vi "Galvo Module_sync.vi"(5 "sample mode":i32(ring)=10178 items=["Finite Samples"=10178, "Continuous Samples"=10123, "Hardware Timed Single Point"=12522], 7 "Action":T23(ring)=enum."Init: Calc scan pattern", 8 "error in (no error)":errorcluster, 10 "System Parameters":T1={"Optical Parameters"={"Obj. Focal Length [mm]"=45.0, "Scan Lens EFL[mm]"=60.0, "Tube Lens EFL[mm]"=180.0, "Galvo V Range (+/-)"=10.0, "Galvo Max Half Angle [Deg]"=19.0, "Max Galvo Range[%]"=0.0}, "Vibratome"={"Pre Cut Dwell [s]"=0.0, "Blade Frequency [RPM]"=0, "Slice Speed [mm/s]"=0.0, "Post Cut Dwell [s]"=0.0, "Ramp Time [s]"=0.0, "Start X [mm]"=0.0, "Start Y [mm]"=0.0, "Slice Length [mm]"=0.0, "Slice Axis"=enum."Y Axis", "Controller VISA Ref"="COM4", "Blade Frequency [Hz]"=0, "Analog Out Channel"="GalvoCtrl/ao0,GalvoCtrl/ao1", "Pixel Clock Source"="/GalvoCtrl/PFI0", "Vib version"=enum."Vibratome1"}, "Table Stages"={"X Stage"={"Position"=0.0, "Is.Enabled?"=FALSE, "Is.Connected?"=FALSE, "Device SN"="45876539", "AccelerationMaximum"=0.0, "VelocityMaximum"=0.0, "Acceleration"=0.0, "Velocity"=0.0, "waitTimeout (ms)"=0, "Model"=enum."None", "Is.Homed?"=FALSE, "MOVE"=FALSE}, "Y Stage"={"Position"=0.0, "Is.Enabled?"=FALSE, "Is.Connected?"=FALSE, "Device SN"="45876539", "AccelerationMaximum"=0.0, "VelocityMaximum"=0.0, "Acceleration"=0.0, "Velocity"=0.0, "waitTimeout (ms)"=0, "Model"=enum."None", "Is.Homed?"=FALSE, "MOVE"=FALSE}, "Z Stage"={"Position"=0.0, "Is.Enabled?"=FALSE, "Is.Connected?"=FALSE, "Device SN"="45876539", "AccelerationMaximum"=0.0, "VelocityMaximum"=0.0, "Acceleration"=0.0, "Velocity"=0.0, "waitTimeout (ms)"=0, "Model"=enum."None", "Is.Homed?"=FALSE, "MOVE"=FALSE}, "Attenuator"={"Position"=0.0, "Is.Enabled?"=FALSE, "Is.Connected?"=FALSE, "Device SN"="45876539", "AccelerationMaximum"=0.0, "VelocityMaximum"=0.0, "Acceleration"=0.0, "Velocity"=0.0, "waitTimeout (ms)"=0, "Model"=enum."None", "Is.Homed?"=FALSE, "MOVE"=FALSE}}, "Imaging Parameter"={"Raster Scan Direction"=enum."Uni Directional", "Pixel Dwell Time [Clock Cycles]"=1, "Flyback Time [Clock Cycles]"=10, "XY Center [um]"={"X"=1.0, "Y"=1.0}, "Pixel Step Size [um] X"=50.0, "XY Image Size"=enum."256 x 256", "Custom"=TRUE, "Custom Size"={"X"=10, "Y"=10}, "Line Averages"=1, "Pixel Step Size [um] Y"=0.0}, "Galvo HW Parameters"={"Analog Out Channel"="GalvoCtrl/ao0,GalvoCtrl/ao1", "Min Voltage"=-10.0, "Max Voltage"=10.0, "Pixel Clock Source"="/GalvoCtrl/PFI0", "Sample Rate"=1000.0, "Line Clock Out Ch"="GalvoCtrl/port0/line0", "2P ready check"="GalvoCtrl/port0/line0"}, "Alazar parameters"={"Trigger Settings"={"General Trigger Settings"={"Trigger Operation"=0, "Coupling ID"=2, "Range ID"=2, "Delay"=0, "Timeout Ticks"=0, "Mode"=1, "Parameter"=1}, "Trigger Engine 1"={"Trigger Engine"=0, "Source"=2, "Slope"=1, "Level"=140}, "Trigger Engine 2"={"Trigger Engine"=1000, "Source"=4294967295, "Slope"=1, "Level"=2048}}, "Device ID"={"System ID"=1, "Board ID"=1}, "Ch A Input Control"={"Channel"=1, "Coupling"=2, "Range"=10, "Impedance"=2}, "Ch B Input Control"={"Channel"=2, "Coupling"=2, "Range"=10, "Impedance"=2}, "Acq Settings"={"Record Length"=1440, "Offset"=0, "Records Per Buffer"=2048, "Records Count (Records/Acq)"=2147483647, "Window Type"=1, "Footer"=0, "Samples per record"=2048, "Output Format"=257}, "Capture Clock"={"Sample Rate"=100, "Decimation"=0, "Source"=2, "Edge"=0}}, "Mosaic Paramter"={"X Axis"={"Start [mm]"=0.0, "Steps [pts]"=0.0, "End [mm]"=0.0}, "Y Axis"={"Start [mm]"=0.0, "Steps [pts]"=0.0, "End [mm]"=0.0}, "Scan Pattern"=enum."Uni-directional", "Overlap Options"={"Overlap Type"=enum."No Overlap", "Percent Overlap"=0, "Justify"=enum."Start"}}, "Manual Controls"={"Data Path"=path "", "Save parameters"={"start pixel"=45, "#pixels to save"=100}, "Acquisition mode"=enum."Alazar FFT", "PSOCT Channel"=1, "Save data?"=FALSE, "AIP rotation angle"=0.0, "Pause acquisition?"=FALSE, "Outgoing Mail Server (SMTP)"="smtp.gmail.com", "Email"="", "Password"="", "Carrier 1"=enum."Sprint", "phone number 1"="", "Subject"="", "Message"="", "Carrier 2"=enum."Sprint", "phone number 2"="", "Check boundary?"=FALSE, "Threshold"=0.0, "Outputs for GPU FFT"=enum."Amp + Phase diff"}, "Z stage setting"={"first cut height(mm)"=45.85, "slice thickness[um]"=[], "#repetitions"=111, "image thickness(um)"=[], "#cycles per repetition"=0, "First image height(mm)"=2.1, "Block?"=[], "Z0"=0.0, "fixed Z0?"=FALSE}, "Attenuator"={"Power after Objective (recalibrate every 6 month)"=[]}} {"Manual Controls"."PSOCT Channel" items=["A"=1, "B"=2, "A + B"=3, "C"=4, "A + C"=5, "A + B"=6, "D"=8, "A + D"=9, "B + D"=10, "C + D"=12, "A + B + C + D"=15]; "Alazar parameters"."Capture Clock"."Edge" items=["Rising", "Falling"]; "Alazar parameters"."Capture Clock"."Source" items=["Internal"=1, "Fast External"=2, "Medium External"=3, "Slow External"=4, "External AC"=5, "External DC"=6, "External 10MHz"=7]; "Alazar parameters"."Acq Settings"."Output Format" items=["Float Log"=11, "Float Amp"=10, "U16_LOG"=1, "U16_AMP2"=257, "Real"=3, "Imag"=4]; "Alazar parameters"."Acq Settings"."Footer" items=["FOOTER_NONE", "FOOTER_NPT"]; "Alazar parameters"."Acq Settings"."Window Type" items=["DSP_WINDOW_NONE", "DSP_WINDOW_HANNING", "DSP_WINDOW_HAMMING", "DSP_WINDOW_BLACKMAN", "DSP_WINDOW_BLACKMAN_HARRIS", "DSP_WINDOW_BARTLETT"]; "Alazar parameters"."Ch B Input Control"."Channel" items=["A"=1, "B"=2, "C"=4, "D"=8]; "Alazar parameters"."Ch B Input Control"."Coupling" items=["AC"=1, "DC"=2]; "Alazar parameters"."Ch B Input Control"."Range" items=["20 mV"=1, "40 mV"=2, "50 mV"=3, "80 mV"=4, "100 mV"=5, "200 mV"=6, "400 mV"=7, "500 mV"=8, "800 mV"=9, "1 V"=10, "1.25 V"=33, "2 V"=11, "4 V"=12, "5 V"=13, "8 V"=14, "10 V"=15, "20 V"=16]; "Alazar parameters"."Ch B Input Control"."Impedance" items=["1 MOhm"=1, "50 Ohm"=2, ""=0]; "Alazar parameters"."Ch A Input Control"."Channel" items=["A"=1, "B"=2, "C"=4, "D"=8]; "Alazar parameters"."Ch A Input Control"."Coupling" items=["AC"=1, "DC"=2]; "Alazar parameters"."Ch A Input Control"."Range" items=["20 mV"=1, "40 mV"=2, "50 mV"=3, "80 mV"=4, "100 mV"=5, "200 mV"=6, "400 mV"=7, "500 mV"=8, "800 mV"=9, "1 V"=10, "1.25 V"=33, "2 V"=11, "4 V"=12, "5 V"=13, "8 V"=14, "10 V"=15, "20 V"=16]; "Alazar parameters"."Ch A Input Control"."Impedance" items=["1 MOhm"=1, "50 Ohm"=2, ""=0]; "Alazar parameters"."Trigger Settings"."General Trigger Settings"."Trigger Operation" items=["J", "K", "J OR K", "J AND K", "J XOR K", "J AND NOT K", "NOT J AND K"]; "Alazar parameters"."Trigger Settings"."General Trigger Settings"."Coupling ID" items=["AC"=1, "DC"=2]; "Alazar parameters"."Trigger Settings"."General Trigger Settings"."Range ID" items=["5 V", "1 V", "TTL"]; "Alazar parameters"."Trigger Settings"."Trigger Engine 1"."Trigger Engine" items=["J", "K"]; "Alazar parameters"."Trigger Settings"."Trigger Engine 1"."Source" items=["A", "B", "External", "Disable", "C", "D"]; "Alazar parameters"."Trigger Settings"."Trigger Engine 1"."Slope" items=["Positive"=1, "Negative"=2]; "Alazar parameters"."Trigger Settings"."Trigger Engine 2"."Trigger Engine" items=["J", "K"]; "Alazar parameters"."Trigger Settings"."Trigger Engine 2"."Source" items=["A", "B", "External", "Disable", "C", "D"]; "Alazar parameters"."Trigger Settings"."Trigger Engine 2"."Slope" items=["Positive"=1, "Negative"=2]; "Imaging Parameter"."Pixel Step Size [um] Y" min=0.0 max=100.0 step=0.01; "Imaging Parameter"."Line Averages" min=1 max=30 step=1; "Imaging Parameter"."Flyback Time [Clock Cycles]" max=10 step=1; "Imaging Parameter"."Pixel Step Size [um] X" min=0.0 max=100.0 step=0.01; "Imaging Parameter"."Custom Size"."Y" min=1 max=30 step=1; "Imaging Parameter"."Custom Size"."X" min=1 max=30 step=1; "Imaging Parameter"."XY Center [um]"."Y" min=1.0 max=30.0 step=1.0; "Imaging Parameter"."XY Center [um]"."X" min=1.0 max=30.0 step=1.0; "Imaging Parameter"."Pixel Dwell Time [Clock Cycles]" max=10 step=1}) -> (0 "error out":errorcluster, 1 "task done?":bool)   [LabVIEW 2018]
uses:
  Controls/System Parameters.ctl
  Controls/Optical Parameters.ctl
  Controls/Vibratome Parameters.ctl
  type defines/vibratome.ctl
  Controls/Translation Stage Parameters.ctl
  Hardware Mfg/Thorlabs Translation Stages/Controls/Translation Stage Cluster.ctl
  Controls/Translation Stage Types.ctl
  Controls/Imaging Parameters.ctl
  Controls/Scan Direction.ctl
  type defines/Alazar parameters.ctl
  Hardware Mfg/AlazarTech SDK/Controls/General Trigger Settings.ctl
  Hardware Mfg/AlazarTech SDK/Controls/Trigger Engine Controls.ctl
  Hardware Mfg/AlazarTech SDK/Controls/Alazar Device ID.ctl
  Hardware Mfg/AlazarTech SDK/Controls/Channel Input Controls.ctl
  Hardware Mfg/AlazarTech SDK/Controls/Alazar Acquisition Settings.ctl
  Hardware Mfg/AlazarTech SDK/Controls/Clock Controls.ctl
  type defines/Manual Controls.ctl
  type defines/FFT parameters.ctl
  type defines/FFT mode.ctl
  type defines/GPU FFT outputs.ctl
  type defines/Vibratome Param.ctl
  type defines/attenuator.ctl
  <vilib>/DAQmx/write.llb/DAQmx Write (Digital 1D U32 1Chan NSamp).vi
  <vilib>/DAQmx/write.llb/DAQmx Write (Analog 2D DBL NChan NSamp).vi
  <vilib>/DAQmx/create/channels.llb/DAQmx Create Channel (CO-Pulse Generation-Time).vi
  <vilib>/DAQmx/create/channels.llb/DAQmx Create Channel (AO-Voltage-Basic).vi
  <vilib>/DAQmx/configure/timing.llb/DAQmx Timing (Sample Clock).vi
  <vilib>/DAQmx/create/channels.llb/DAQmx Create Channel (DO-Digital Output).vi
  <vilib>/DAQmx/configure/trigger.llb/DAQmx Start Trigger (Digital Edge).vi
  <vilib>/DAQmx/miscellaneous.llb/DAQmx Fill In Error Info.vi
  <resource>/objmgr/daqmx.rc
panel:
  # "X"
  # "X"
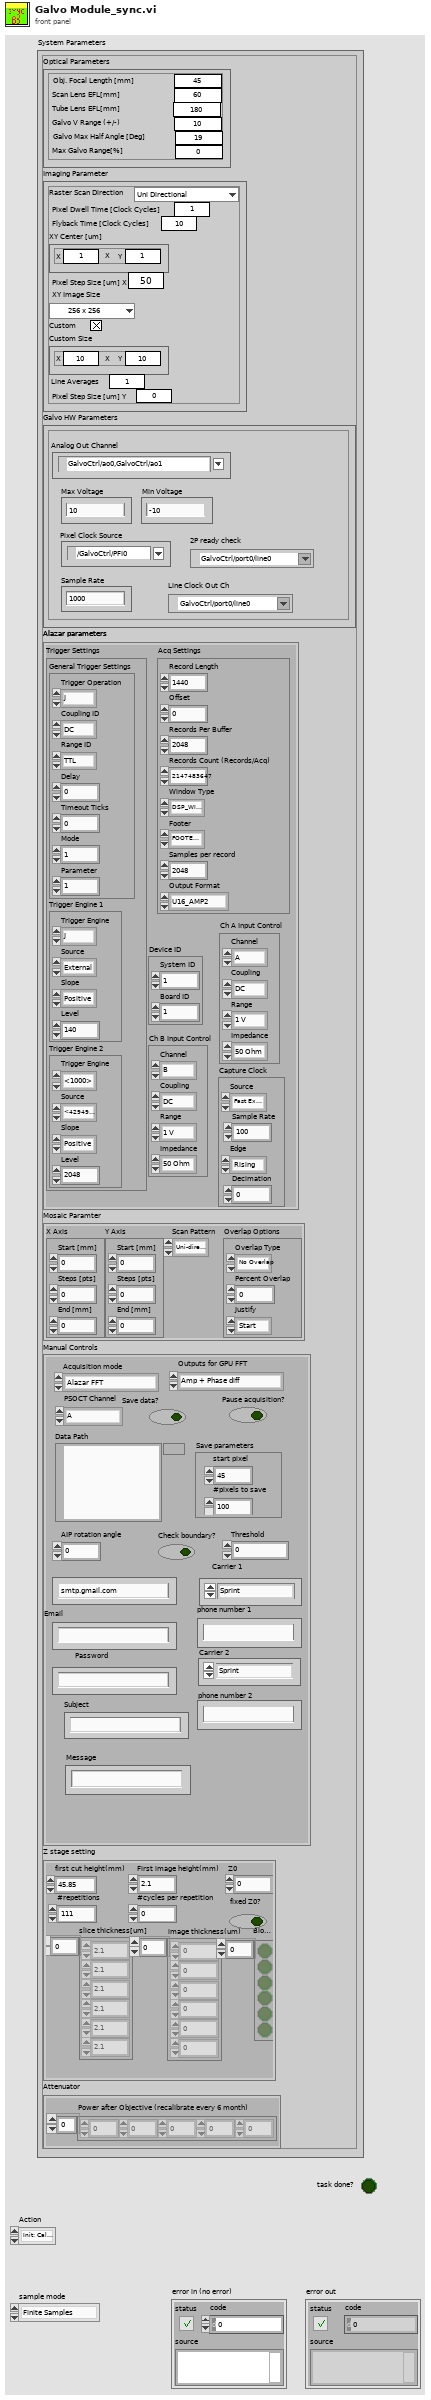
[diagram p1: front panel]
types:
  T1 = typedef "System Parameters.ctl" = cluster{"Optical Parameters":T2, "Vibratome":T3, "Table Stages":T5, "Imaging Parameter":T8, "Galvo HW Parameters":cluster{"Analog Out Channel":tag, "Min Voltage":dbl, "Max Voltage":dbl, "Pixel Clock Source":tag, "Sample Rate":dbl, "Line Clock Out Ch":tag, "2P ready check":tag}, "Alazar parameters":T10, "Mosaic Paramter":cluster{"X Axis":cluster{"Start [mm]":dbl, "Steps [pts]":dbl, "End [mm]":dbl}, "Y Axis":cluster{"Start [mm]":dbl, "Steps [pts]":dbl, "End [mm]":dbl}, "Scan Pattern":enum16{"Uni-directional", "Bi-Directional", "Spiral Out", "Spiral In"}, "Overlap Options":cluster{"Overlap Type":enum16{"No Overlap", "X Only", "Y Only", "X and Y"}, "Percent Overlap":u8, "Justify":enum16{"Start", "Center", "End"}}}, "Manual Controls":T17, "Z stage setting":T21, "Attenuator":T22}
  T2 = typedef "Optical Parameters.ctl" = cluster{"Obj. Focal Length [mm]":dbl, "Scan Lens EFL[mm]":dbl, "Tube Lens EFL[mm]":dbl, "Galvo V Range (+/-)":dbl, "Galvo Max Half Angle [Deg]":dbl, "Max Galvo Range[%]":dbl}
  T3 = typedef "Vibratome Parameters.ctl" = cluster{"Pre Cut Dwell [s]":dbl, "Blade Frequency [RPM]":u16, "Slice Speed [mm/s]":dbl, "Post Cut Dwell [s]":dbl, "Ramp Time [s]":dbl, "Start X [mm]":dbl, "Start Y [mm]":dbl, "Slice Length [mm]":dbl, "Slice Axis":enum16{"X Axis", "Y Axis", "Z Axis"}, "Controller VISA Ref":refnum<visa-resource-name>, "Blade Frequency [Hz]":u16, "Analog Out Channel":tag, "Pixel Clock Source":tag, "Vib version":T4}
  T4 = typedef "vibratome.ctl" = enum16{"Vibratome1", "Vibratome3"}
  T5 = typedef "Translation Stage Parameters.ctl" = cluster{"X Stage":T6, "Y Stage":T6, "Z Stage":T6, "Attenuator":T6}
  T6 = typedef "Translation Stage Cluster.ctl" = cluster{"Position":dbl, "Is.Enabled?":bool, "Is.Connected?":bool, "Device SN":string, "AccelerationMaximum":dbl, "VelocityMaximum":dbl, "Acceleration":dbl, "Velocity":dbl, "waitTimeout (ms)":i32, "Model":T7, "Is.Homed?":bool, "MOVE":bool}
  T7 = typedef "Translation Stage Types.ctl" = enum16{"None", "Thorlabs LTS", "Thorlabs MLJ"}
  T8 = typedef "Imaging Parameters.ctl" = cluster{"Raster Scan Direction":T9, "Pixel Dwell Time [Clock Cycles]":u16, "Flyback Time [Clock Cycles]":u16, "XY Center [um]":cluster{"X":dbl, "Y":dbl}, "Pixel Step Size [um] X":dbl, "XY Image Size":enum16{"32 x 32", "64 x 64", "128 x 128", "256 x 256", "512 x 512", "1024 x 1024", "2048 x 2048"}, "Custom":bool, "Custom Size":cluster{"X":u16, "Y":u16}, "Line Averages":u8, "Pixel Step Size [um] Y":dbl}
  T9 = typedef "Scan Direction.ctl" = enum16{"Uni Directional", "Bi Directional", "None"}
  T10 = typedef "Alazar parameters.ctl" = cluster{"Trigger Settings":cluster{"General Trigger Settings":T11, "Trigger Engine 1":T12, "Trigger Engine 2":T12}, "Device ID":T13, "Ch A Input Control":T14, "Ch B Input Control":T14, "Acq Settings":T15, "Capture Clock":T16}
  T11 = typedef "General Trigger Settings.ctl" = cluster{"Trigger Operation":u32, "Coupling ID":u32, "Range ID":u32, "Delay":u32, "Timeout Ticks":u32, "Mode":u32, "Parameter":u32}
  T12 = typedef "Trigger Engine Controls.ctl" = cluster{"Trigger Engine":u32, "Source":u32, "Slope":u32, "Level":u32}
  T13 = typedef "Alazar Device ID.ctl" = cluster{"System ID":u32, "Board ID":u32}
  T14 = typedef "Channel Input Controls.ctl" = cluster{"Channel":u8, "Coupling":u32, "Range":u32, "Impedance":u32}
  T15 = typedef "Alazar Acquisition Settings.ctl" = cluster{"Record Length":u32, "Offset":u32, "Records Per Buffer":u32, "Records Count (Records/Acq)":u32, "Window Type":u32, "Footer":u32, "Samples per record":u32, "Output Format":u32}
  T16 = typedef "Clock Controls.ctl" = cluster{"Sample Rate":u32, "Decimation":u32, "Source":u32, "Edge":u32}
  T17 = typedef "Manual Controls.ctl" = cluster{"Data Path":path, "Save parameters":T18, "Acquisition mode":T19, "PSOCT Channel":u32, "Save data?":bool, "AIP rotation angle":dbl, "Pause acquisition?":bool, "Outgoing Mail Server (SMTP)":string, "Email":string, "Password":string, "Carrier 1":enum16{"T-Mobile", "AT&T", "Verizon", "Sprint"}, "phone number 1":string, "Subject":string, "Message":string, "Carrier 2":enum16{"T-Mobile", "AT&T", "Verizon", "Sprint"}, "phone number 2":string, "Check boundary?":bool, "Threshold":sgl, "Outputs for GPU FFT":T20}
  T18 = typedef "FFT parameters.ctl" = cluster{"start pixel":i32, "#pixels to save":i32}
  T19 = typedef "FFT mode.ctl" = enum16{"ThorOCT B line", "ThorOCT Spectral", "ThorOCT FFT", "Alazar B line", "Alazar FFT", "GPU FFT", "Alazar Spectral", "Simulation", "auto adjust focus", "Save all"}
  T20 = typedef "GPU FFT outputs.ctl" = enum16{"Amp + Phase diff", "Amp + Phase", "Amp only"}
  T21 = typedef "Vibratome Param.ctl" = cluster{"first cut height(mm)":dbl, "slice thickness[um]":dbl[], "#repetitions":u16, "image thickness(um)":dbl[], "#cycles per repetition":u16, "First image height(mm)":dbl, "Block?":bool[], "Z0":dbl, "fixed Z0?":bool}
  T22 = typedef "attenuator.ctl" = cluster{"Power after Objective (recalibrate every 6 month)":dbl[]}
  T23 = enum16{"Configure channels", "Write Scan Pattern", "Start Galvo Task", "Is Task Done?", "Stop Galvo", "Uninit", "Init: Calc scan pattern"}
  T24 = cluster{"Analog Out Channel":tag, "Min Voltage":dbl, "Max Voltage":dbl, "Pixel Clock Source":tag, "Sample Rate":dbl, "Line Clock Out Ch":tag, "2P ready check":tag}
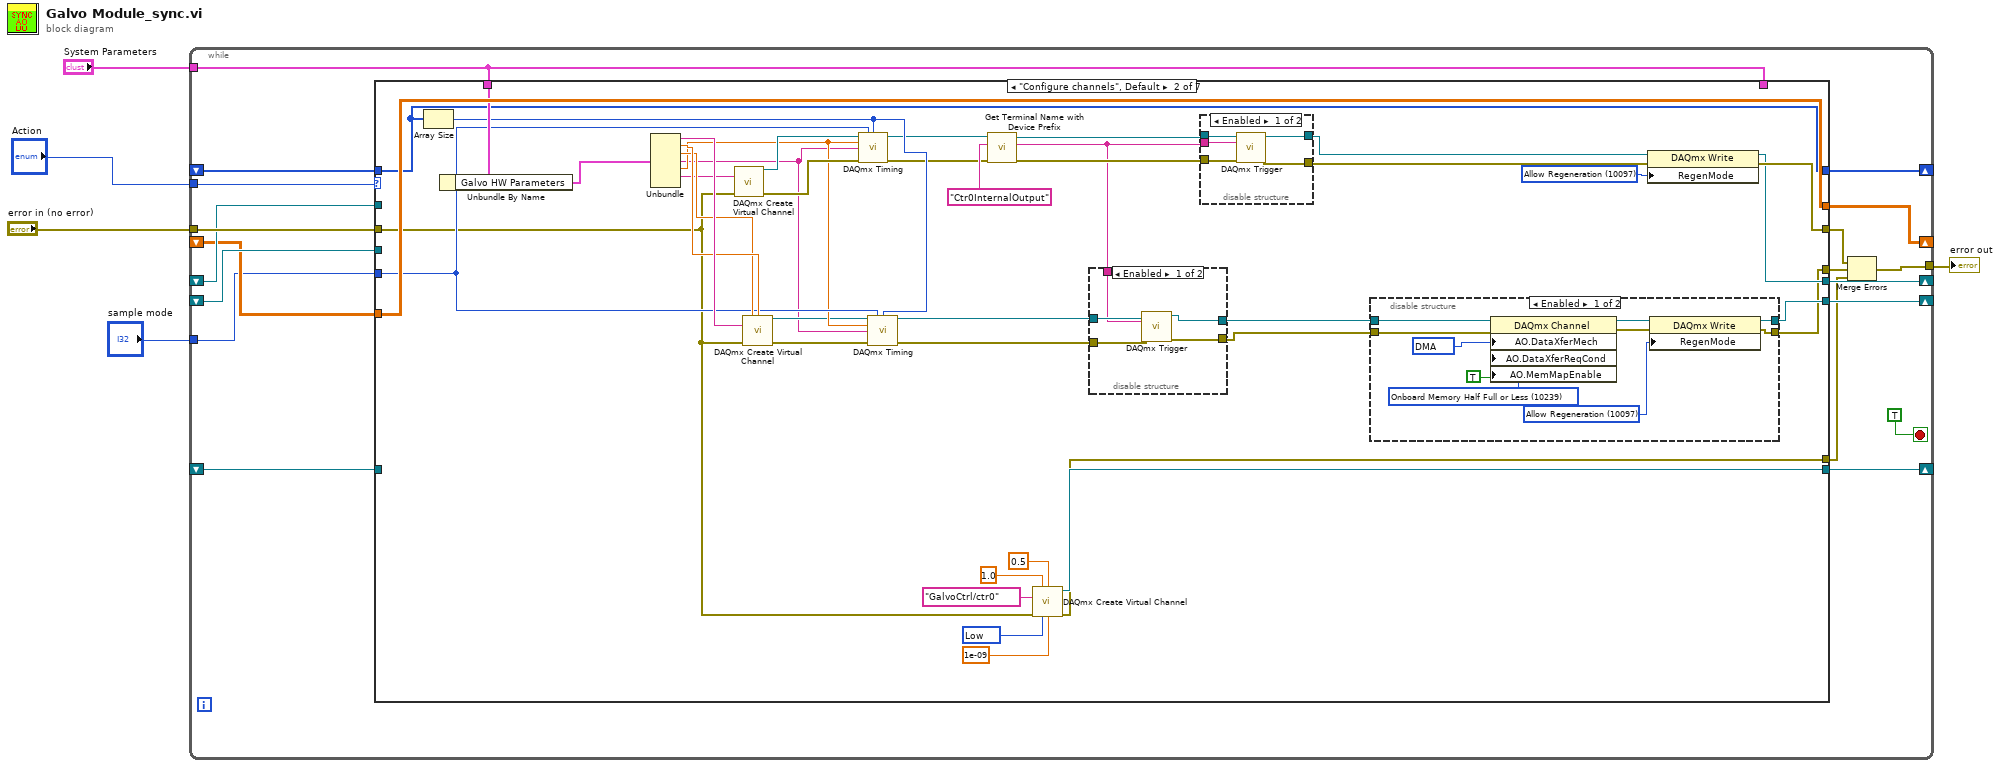
[diagram p0: block diagram]
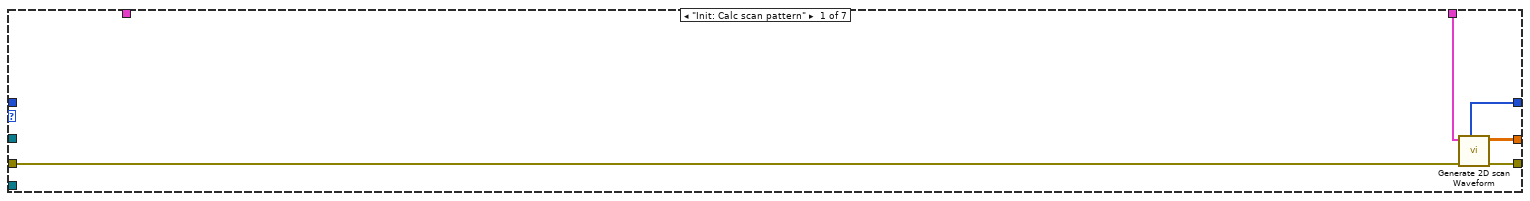
[diagram p2: hidden frame]
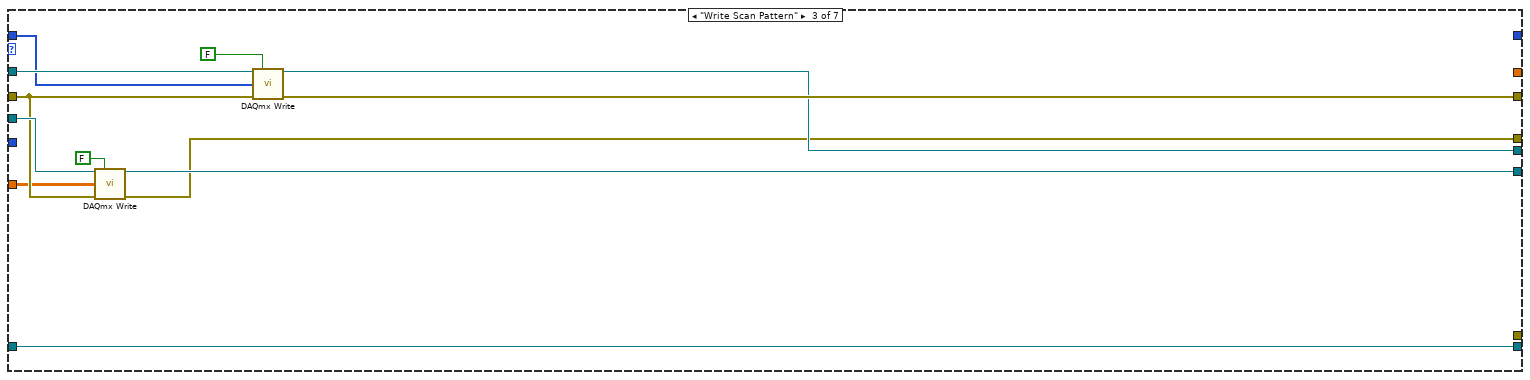
[diagram p6: hidden frame]
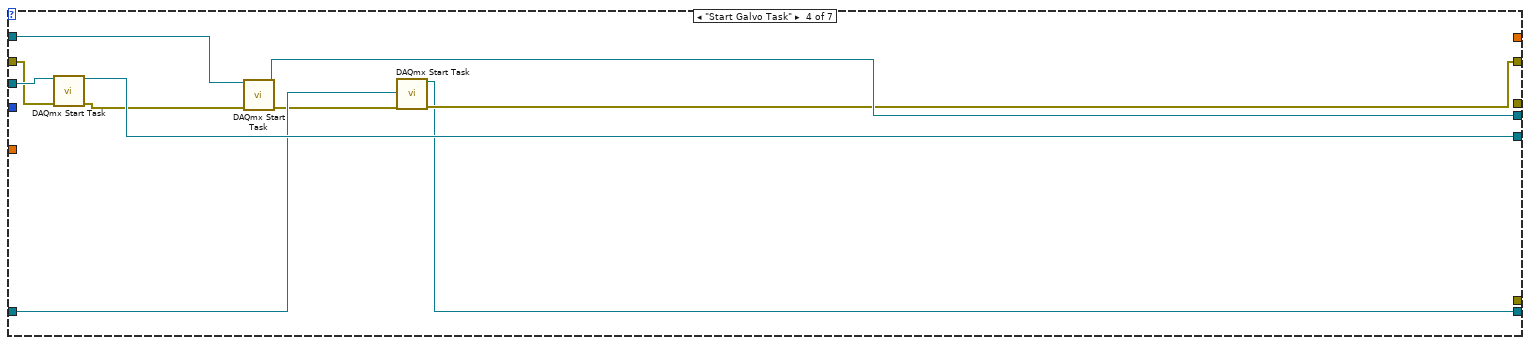
[diagram p7: hidden frame]
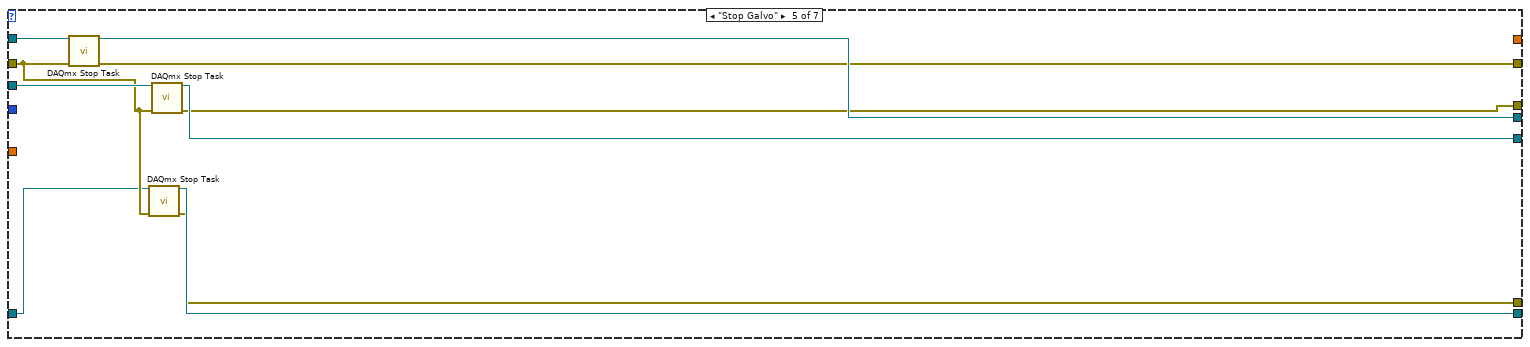
[diagram p8: hidden frame]
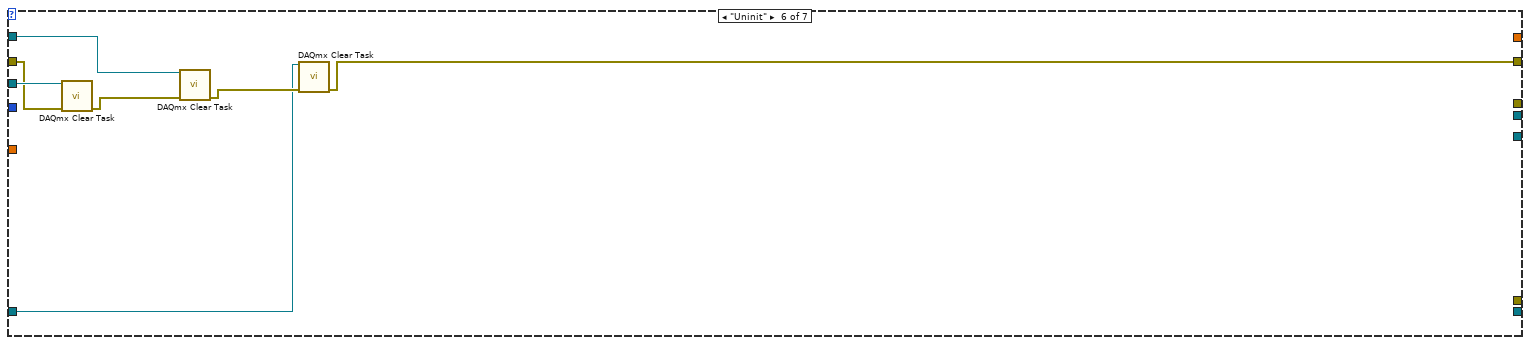
[diagram p9: hidden frame]
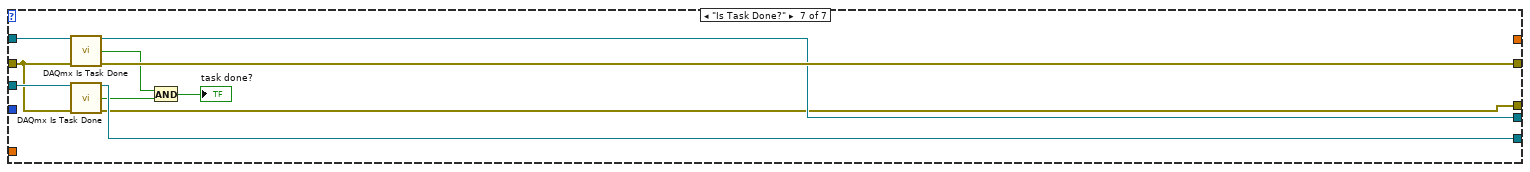
[diagram p10: hidden frame]
diagram:
  n1 = while {
    tunnel: "Action" -> [w24]
    shift-right: [w23] -> _
    shift-left: _ -> [w22]
    tunnel: [w19] -> w4
    tunnel: "error in (no error)" -> [w21]
    shift-right: [w17] -> _
    shift-left: _ -> [w16]
    shift-right: [w15] -> _
    shift-left: _ -> [w14]
    tunnel: "sample mode" -> [w13]
    tunnel: "System Parameters" -> [w11]
    shift-right: [w10] -> _
    shift-left: _ -> [w9]
    shift-right: [w8] -> _
    shift-left: _ -> [w7]
    stop <- TRUE stop-if-true
    n2 = case shown="\"Configure channels\", Default" w24 {
      tunnel: [_ w67 w102 w117 w127 _ w144] -> w23
      tunnel: w22 -> [_ _ w108 w118 w128 w135 w145]
      tunnel: w21 -> [w27 w46 w107 w114 w122 w133 w136]
      tunnel: [w28 w63 w106 w110 w124 w130 w141] -> w18
      tunnel: [_ w62 w104 w115 w125 _ w138] -> w17
      tunnel: w16 -> [_ _ w103 w116 w126 w134 w142]
      tunnel: [w29 w61 _ _ _ _ _] -> w15
      tunnel: w14 -> [_ w61 w101 _ _ _ _]
      tunnel: w13 -> [_ w57 _ _ _ _ _]
      tunnel: [_ w60 w100 _ w123 _ w137] -> w12
      tunnel: w11 -> [w26 _ _ _ _ _ _]
      tunnel: w11 -> [_ w59 _ _ _ _ _]
      tunnel: [w25 w54 _ _ _ _ _] -> w10
      tunnel: w9 -> [_ w54 w99 _ _ _ _]
      tunnel: [_ w38 w97 w109 w120 _ _] -> w8
      tunnel: w7 -> [_ _ w97 w112 w121 w129 _]
      tunnel: [_ w37 _ _ w119 _ _] -> w6
      frame "Init: Calc scan pattern" {
        n3 = call "Generate 2D scan Waveform.vi"("error in (no error)"=w27, "System Parameters [In]"=w26) -> ("error out"=w28:errorcluster, "XY"=w29:dbl[][], "DO"=w25:u32[])  [unwired: 3 in, 4 out]
      }
      frame "Configure channels", Default {
        w30 = 10097 items=["Allow Regeneration"=10097, "Do Not Allow Regeneration"=10158] ("RegenMode")
        w51 = 10214 items=["High"=10192, "Low"=10214] ("Idle State")
        n4 = Array Size(array=w54) -> (size(s)=w56:i32)
        n5 = Unbundle By Name(w59) -> ("Galvo HW Parameters"=w58:T24)
        n6 = Unbundle(w58) -> ("Analog Out Channel"=w70:tag, "Min Voltage"=w69:dbl, "Max Voltage"=w68:dbl, "Pixel Clock Source"=w36:tag, "Sample Rate"=w55:dbl, "Line Clock Out Ch"=w66:tag)  [unwired: 1 out]
        n7 = call-poly <vilib>:"DAQmx Create Virtual Channel.vi"("lines"=w66, "error in"=w46) -> ("task out"=w64:refnum<k21>, "error out"=w65:errorcluster)  [unwired: 12 in]
        n8 = call-poly <vilib>:"DAQmx Create Virtual Channel.vi"("maximum value"=w68, "minimum value"=w69, "physical channels"=w70, "error in"=w46) -> ("task out"=w53:refnum<k21>, "error out"=w52:errorcluster)  [unwired: 10 in]
        n9 = call-poly <vilib>:"DAQmx Timing.vi"("task/channels in"=w64, "sample mode"=w57, "samples per channel"=w56, "rate"=w55, "source"=w36, "error in"=w65) -> ("task out"=w43:refnum<k21>, "error out"=w44:errorcluster)  [unwired: 8 in]
        n10 = call-poly <vilib>:"DAQmx Timing.vi"("task/channels in"=w53, "sample mode"=w57, "samples per channel"=w56, "rate"=w55, "source"=w36, "error in"=w52) -> ("task out"=w40:refnum<k21>, "error out"=w42:errorcluster)  [unwired: 8 in]
        n11 = call "Get Terminal Name with Device Prefix.vi"("error in (no error)"=w44, "Local Terminal Name"="Ctr0InternalOutput" ("terminal"), "task/channels in"=w43) -> ("error out"=w35:errorcluster, "Terminal Name with Device Prefix"=w31:tag, "task out"=w34:refnum<k21>)  [unwired: 1 in, 5 out]
        n12 = call-poly <vilib>:"DAQmx Create Virtual Channel.vi"("high time"=1.0 ("High Time"), "low time"=0.5 ("Low Time"), "counter"=tag "GalvoCtrl/ctr0" ("Counter(s)"), "error in"=w46, "idle state"=w51, "initial delay"=1e-09 ("Initial Delay")) -> ("task out"=w38:refnum<k21>, "error out"=w37:errorcluster)  [unwired: 3 in, 5 out]
        n13 = disable-structure shown="Enabled" {
          disable-tunnel: w42 -> [w82 w83]
          disable-tunnel: [w81 w83] -> w41
          disable-tunnel: w40 -> [w80 w84]
          disable-tunnel: [w79 w84] -> w39
          disable-tunnel: w31 -> [w78 _]
          frame Enabled {
            n14 = call-poly <vilib>:"DAQmx Trigger.vi"("task/channels in"=w80, "source"=w78, "error in"=w82) -> ("task out"=w79:refnum<k21>, "error out"=w81:errorcluster)  [unwired: 2 in, 9 out]
          }
          frame Disabled {
          }
        }
        n15 = disable-structure shown="Enabled" {
          disable-tunnel: w35 -> [w75 w77]
          disable-tunnel: w34 -> [w74 w76]
          disable-tunnel: [w73 w76] -> w33
          disable-tunnel: [w72 w77] -> w32
          disable-tunnel: w31 -> [w71 _]
          frame Enabled {
            n16 = call-poly <vilib>:"DAQmx Trigger.vi"("task/channels in"=w74, "source"=w71, "error in"=w75) -> ("task out"=w73:refnum<k21>, "error out"=w72:errorcluster)  [unwired: 2 in, 9 out]
          }
          frame Disabled {
          }
        }
        n17 = disable-structure shown="Enabled" {
          disable-tunnel: w41 -> [w94 w95]
          disable-tunnel: w39 -> [w92 w96]
          disable-tunnel: [w88 w95] -> w60
          disable-tunnel: [w85 w96] -> w67
          frame Enabled {
            w86 = 10097 items=["Allow Regeneration"=10097, "Do Not Allow Regeneration"=10158] ("RegenMode")
            w90 = 10239 items=["Onboard Memory Empty"=10235, "Onboard Memory Half Full or Less"=10239, "Onboard Memory Less than Full"=10242] ("AO.DataXferReqCond")
            w91 = 10054 items=["DMA"=10054, "Interrupts"=10204, "Programmed I/O"=10264, "USB Bulk"=12590] ("AO.DataXferMech")
            n18 = property class="DAQmx Channel"(reference=w92, error in=w94, "AO.DataXferMech"=w91, "AO.DataXferReqCond"=w90, "AO.MemMapEnable"=TRUE) -> (reference out=w87:refnum<k21>, error out=w93:errorcluster)
            n19 = property class="DAQmx Write"(reference=w87, error in=w93, "RegenMode"=w86) -> (reference out=w85:refnum<k21>, error out=w88:errorcluster)
          }
          frame Disabled {
          }
        }
        n20 = property class="DAQmx Write"(reference=w33, error in=w32, "RegenMode"=w30) -> (reference out=w62:refnum<k21>, error out=w63:errorcluster)
      }
      frame "Write Scan Pattern" {
        n21 = call-poly <vilib>:"DAQmx Write.vi"("task/channels in"=w108, "auto start"=FALSE, "data"=w101, "error in"=w107) -> ("task out"=w102:refnum<k21>, "error out"=w100:errorcluster)  [unwired: 9 in, 1 out]
        n22 = call-poly <vilib>:"DAQmx Write.vi"("task/channels in"=w103, "auto start"=FALSE, "data"=w99, "error in"=w107) -> ("task out"=w104:refnum<k21>, "error out"=w106:errorcluster)  [unwired: 9 in, 1 out]
      }
      frame "Start Galvo Task" {
        n23 = call <vilib>:"DAQmx Start Task.vi"("task/channels in"=w118, "error in"=w114) -> ("task out"=w117:refnum<k21>, "error out"=w113:errorcluster)  [unwired: 12 in]
        n24 = call <vilib>:"DAQmx Start Task.vi"("task/channels in"=w116, "error in"=w113) -> ("task out"=w115:refnum<k21>, "error out"=w111:errorcluster)  [unwired: 12 in]
        n25 = call <vilib>:"DAQmx Start Task.vi"("task/channels in"=w112, "error in"=w111) -> ("task out"=w109:refnum<k21>, "error out"=w110:errorcluster)  [unwired: 12 in]
      }
      frame "Stop Galvo" {
        n26 = call <vilib>:"DAQmx Stop Task.vi"("task/channels in"=w126, "error in"=w122) -> ("task out"=w125:refnum<k21>, "error out"=w124:errorcluster)  [unwired: 12 in]
        n27 = call <vilib>:"DAQmx Stop Task.vi"("task/channels in"=w121, "error in"=w122) -> ("task out"=w120:refnum<k21>, "error out"=w119:errorcluster)  [unwired: 12 in]
        n28 = call <vilib>:"DAQmx Stop Task.vi"("task/channels in"=w128, "error in"=w122) -> ("task out"=w127:refnum<k21>, "error out"=w123:errorcluster)  [unwired: 12 in]
      }
      frame "Uninit" {
        n29 = call <vilib>:"DAQmx Clear Task.vi"("task in"=w135, "error in"=w133) -> ("error out"=w132:errorcluster)  [unwired: 13 in]
        n30 = call <vilib>:"DAQmx Clear Task.vi"("task in"=w134, "error in"=w132) -> ("error out"=w131:errorcluster)  [unwired: 13 in]
        n31 = call <vilib>:"DAQmx Clear Task.vi"("task in"=w129, "error in"=w131) -> ("error out"=w130:errorcluster)  [unwired: 13 in]
      }
      frame "Is Task Done?" {
        n32 = call <vilib>:"DAQmx Is Task Done.vi"("task/channels in"=w142, "error in"=w136) -> ("task out"=w138:refnum<k21>, "task done?"=w139:bool, "error out"=w141:errorcluster)  [unwired: 11 in]
        n33 = call <vilib>:"DAQmx Is Task Done.vi"("task/channels in"=w145, "error in"=w136) -> ("task out"=w144:refnum<k21>, "task done?"=w143:bool, "error out"=w137:errorcluster)  [unwired: 11 in]
        n34 = And(x=w139, y=w143) -> (x .and. y?=→"task done?":bool)
      }
    }
    n35 = Merge Errors(w18, w12, w6) -> (w19:errorcluster)
  }
  "error out" <- w4
